vi "TrajectoryDashRead.vi"() -> (2 "TrajOrientFF_DegSec":dbl, 3 "TrajOrientDmdDeg":dbl)   [LabVIEW 2023]
uses:
  <vilib>/Rock Robotics/Network Tables/NT Read Number.vi
  <vilib>/Rock Robotics/WPI/ThirdParty/JAS_Junk/TrajLib/Trajectory_Library.lvlib
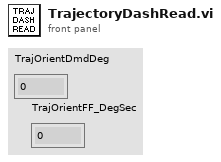
[diagram p1: front panel]
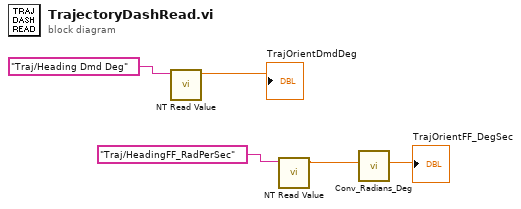
[diagram p0: block diagram]
diagram:
  n1 = call-poly <vilib>:"NT Read Value.vi"("name"="Traj/Heading Dmd Deg" ("Name")) -> ("value"=→"TrajOrientDmdDeg":dbl)  [unwired: 8 in, 2 out]
  n2 = call-poly <vilib>:"NT Read Value.vi"("name"="Traj/HeadingFF_RadPerSec" ("Name")) -> ("value"=w2:dbl)  [unwired: 8 in, 2 out]
  n3 = call <vilib>:"Conv_Radians_Deg.vi"("Radians"=w2) -> ("Degrees"=→"TrajOrientFF_DegSec":dbl)  [unwired: 10 in]
